vi "P1.vi"() -> ()   [LabVIEW 2018]
panel:
  in  "error in (no error)":errorcluster
  out "error out":errorcluster
  out "Image":T1(plugin-control)
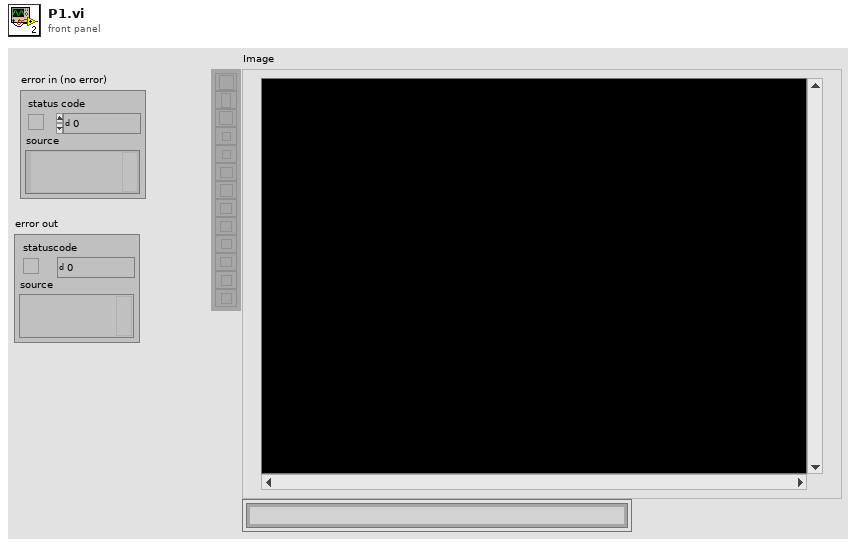
[diagram p1: front panel]
types:
  T1 = typedef "IMAQ Image.ctl" = refnum<image>
  T2 = typedef "Image Type" = u32
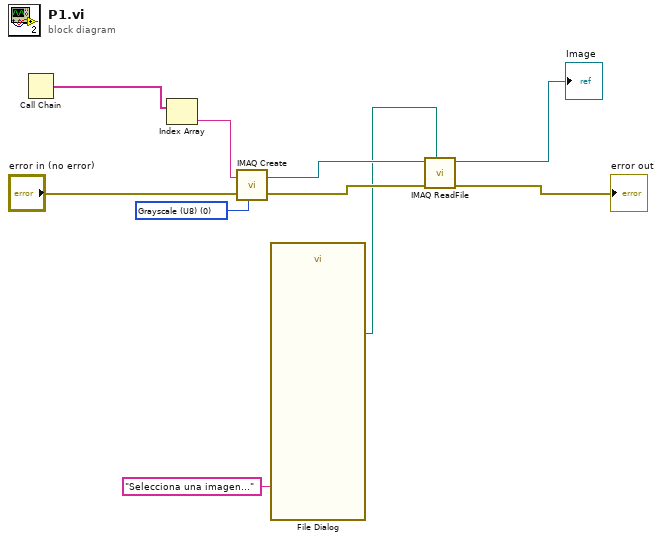
[diagram p0: block diagram]
diagram:
  w1 = T2 0 items=["Grayscale (U8)", "Grayscale (I16)", "Grayscale (SGL)", "Complex (CSG)", "RGB (U32)", "HSL (U32)", "RGB (U64)", "Grayscale (U16)"] ("Image Type")
  n1 = Call Chain() -> (call chain=w7:string[])
  n2 = Index Array "Index Array"(array=w7) -> (element=w6:string)  [unwired: 1 in]
  n3 = call "IMAQ Create"("Image Name"=w6, "Image Type"=w1, "error in (no error)"="error in (no error)") -> ("New Image"=w9:T1, "error out"=w10:errorcluster)  [unwired: 2 in]
  n4 = call "File Dialog"("prompt"="Selecciona una imagen...") -> ("selected path"=w4:path)  [unwired: 11 in, 3 out]
  n5 = call <userlib>:"IMAQ ReadFile.vi"("File Path"=w4, "error in (no error)"=w10, "Image"=w9) -> ("error out"=→"error out":errorcluster, "Image Out"=→"Image":T1)  [unwired: 4 in, 3 out]
